vi "SYST_COMM_GPIB_RDEV_WBL_ID.vi"(0 "VISA IN":refnum<visa-resource-name>, 1 "Block":string, 5 "error in":errorcluster, 7 "ID":i32) -> (14 "VISA Out":refnum<visa-resource-name>, 19 "error out":errorcluster)   [LabVIEW 2018, in "PNA-X.lvlib"]
doc: "SYSTem:COMMunicate:GPIB:RDEVice:WBLock <ID>,<data> \n(Write-only) Same as SYSTem:COMM:GPIB:RDEV:WBIN (above) but the header IS passed along \nto the device. \nUse this command if too many embedded quotes prevent you from using \nSYST:COMM:GPIB:RDEV:WRIT. \nParameters \n<ID> Session identification number that was returned with the OPEN? command. \n<data> Data to be sent to the GPIB pass-through device. See previous command. \nExamples See previous example. \nQuery Syntax Not Applicable \nDefault Not Applicable"
uses:
  PNA-X.lvlib
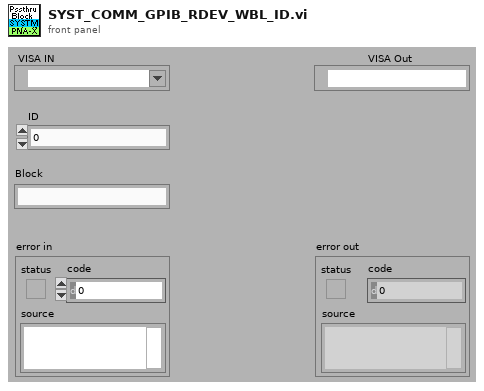
[diagram p1: front panel]
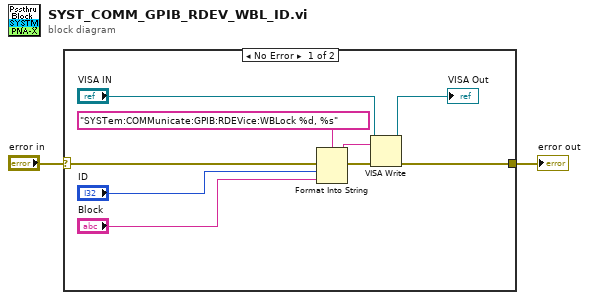
[diagram p0: block diagram]
diagram:
  n1 = case shown="No Error" "error in" {
    selector: "error in" -> [w11 w12]
    tunnel: [w6 w12] -> w1
    frame No Error {
      n2 = Format Into String(format string="SYSTem:COMMunicate:GPIB:RDEVice:WBLock %d, %s" ("Cmdline"), error in=w11, "ID", "Block") -> (resulting string=w9:string, error out=w10:errorcluster)  [unwired: 1 in]
      n3 = VISA Write(VISA resource name="VISA IN", write buffer=w9, error in (no error)=w10) -> (VISA resource name out=→"VISA Out":refnum<visa-resource-name>, error out=w6:errorcluster)  [unwired: 1 out]
    }
    frame Error {
    }
  }
  "error out" <- w1
